vi "Set XY Graph Plot Names.vi"(6 "Reset all":bool, 8 "error in (no error)":errorcluster, 10 "Plot Names []":string[](array[string]), 11 "graph_utilities in":refnum<class "graph_utilities.lvclass">) -> (0 "error out":errorcluster, 3 "graph_utilities out":refnum<class "graph_utilities.lvclass">)   [LabVIEW 2019, in "graph_utilities.lvclass"]
doc: "Set the plot names with option to reset all to \"Plot #\""
uses:
  graph_utilities.lvclass
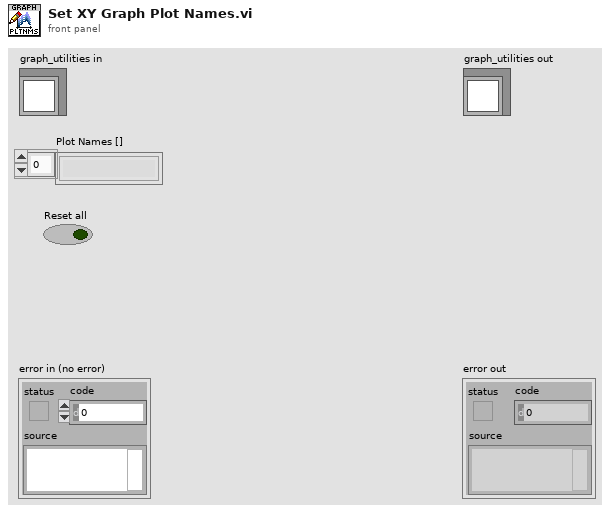
[diagram p1: front panel]
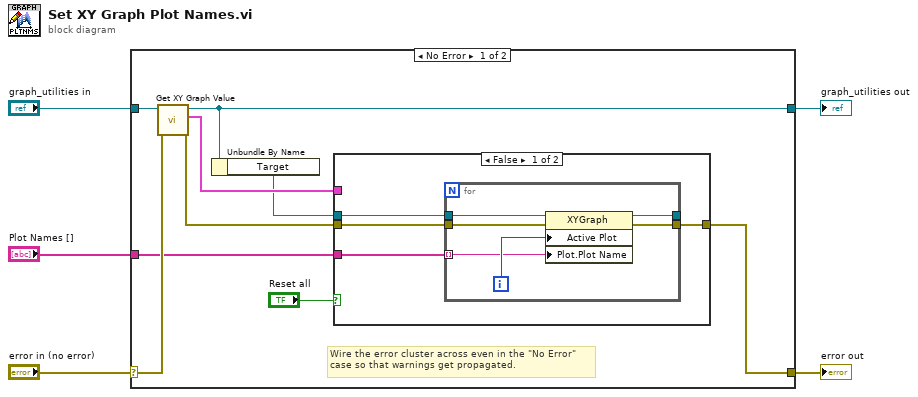
[diagram p0: block diagram]
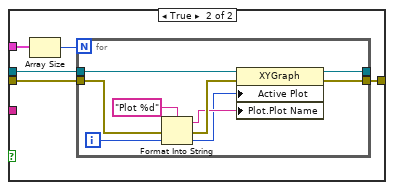
[diagram p2: hidden frame]
diagram:
  n1 = case shown="No Error" "error in (no error)" {
    selector: "error in (no error)" -> [w12 w39]
    tunnel: [w14 w39] -> w4
    tunnel: [w11 w38] -> w2
    tunnel: "graph_utilities in" -> [w13 w38]
    tunnel: "Plot Names []" -> [w6 _]
    frame No Error {
      # "Wire the error cluster across even in the \"No Error\"\ncase so that warnings get propagated."
      n2 = call "Get XY Graph Value.vi"("error in (no error)"=w12, "graph_utilities in"=w13) -> ("error out"=w10:errorcluster, "Value"=w8:cluster{"X":dbl[], "Y":dbl[]}[], "graph_utilities out"=w11:refnum<class "graph_utilities.lvclass">)  [unwired: 7 in]
      n3 = Unbundle By Name(w11) -> ("Target"=w7:refnum<vi>)
      n4 = case shown="False" "Reset all" {
        tunnel: [w18 w29] -> w14
        tunnel: w10 -> [w17 w28]
        tunnel: w6 -> [w16 _]
        tunnel: w7 -> [w15 w27]
        tunnel: w8 -> [_ w25]
        frame False {
          n5 = for {
            tunnel: w17 -> [w24]
            tunnel: [w21] -> w18
            tunnel: w15 -> [w23]
            tunnel: [w22] -> _
            tunnel: w16 -> [w19] mode=indexing
            i -> [w20]
            n6 = property on="Property Node" class="XYGraph"(reference=w23, error in=w24, "Active Plot"=w20, "Plot.Plot Name"=w19) -> (reference out=w22:refnum<vi>, error out=w21:errorcluster)
          }
        }
        frame True {
          n7 = Array Size(array=w25) -> (size(s)=w26:i32)
          n8 = for {
            N: w26 -> [_]
            tunnel: w28 -> [w34]
            tunnel: [w35] -> w29
            tunnel: w27 -> [w37]
            tunnel: [w36] -> _
            i -> [w30]
            n9 = Format Into String(format string="Plot %d", error in=w34, w30) -> (resulting string=w31:string, error out=w33:errorcluster)  [unwired: 1 in]
            n10 = property on="Property Node" class="XYGraph"(reference=w37, error in=w33, "Active Plot"=w30, "Plot.Plot Name"=w31) -> (reference out=w36:refnum<vi>, error out=w35:errorcluster)
          }
        }
      }
    }
    frame Error {
    }
  }
  "error out" <- w4
  "graph_utilities out" <- w2
